vi "niFpga wdp fft sim main frame based.vi"(0 "real data in":fxp<+/-,8,1>[](array[numeric])=[0.0, 0.0], 5 "imaginary data in":fxp<+/-,8,1>[](array[numeric])=[0.0, 0.0], 9 "input frame start":bool, 12 "enable":bool) -> (3 "data indices":u16[](array[numeric]), 4 "real data out":fxp<+/-,19,2>[](array[numeric]), 6 "imaginary data out":fxp<+/-,19,2>[](array[numeric]), 10 "output valid":bool, 14 "ready for frame":bool, 15 "output frame start":bool)   [LabVIEW 2017]
uses:
  <vilib>/rvi/Analysis/measure/FFT/config/niFpgaFFTSettings.ctl
  <vilib>/rvi/Analysis/common/niLvFpgaMspClockRate.ctl
  <vilib>/rvi/Analysis/measure/FFT/config/niFpgaFFTIOPattern.ctl
  <vilib>/rvi/Analysis/measure/FFT/config/niFpgaFFTScalingScheme.ctl
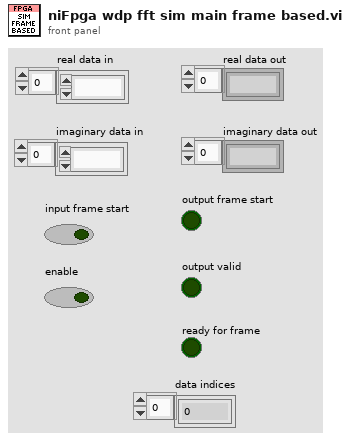
[diagram p1: front panel]
types:
  T1 = typedef "niFpgaFFTSettings.ctl" = cluster{"Number of stages":u8, "Forward?":bool, "adapt to source":bool, "Output word length":u32, "Output integer word length":i32, "Architecture":enum16{"Outside SCTL", "Inside SCTL - Burst", "Inside SCTL - Streaming"}, "input wl":u32, "input iwl":i32, "overflow?":bool, "input sign":enum32{"Signed", "Unsigned"}, "use sim models?":bool, "clock rate":T2, "pattern":T3, "mode":enum16{"Normal", "WDP"}, "scaling scheme":T4, "show enable?":bool}
  T2 = typedef "niLvFpgaMspClockRate.ctl" = enum16{"Default", "Medium", "High"}
  T3 = typedef "niFpgaFFTIOPattern.ctl" = enum16{"CI/CO", "CI/DO", "DI/CO"}
  T4 = typedef "niFpgaFFTScalingScheme.ctl" = enum16{"Unscaled", "Scaled"}
  T5 = typedef "niFpga wdp fft sim model config.ctl" = cluster{"number of stages":i32, "number of spc":i32, "Forward?":bool, "scaling scheme":T4, "internal input type":T6, "tf type":T6, "extra delay":u16, "output shift bits":i16, "reset length":u32, "input shift bits":i16, "pattern":T3}
  T6 = typedef "LVFixedPointRepBitsTypeDef.ctl" = cluster{"Signed":bool, "Word Length":u32, "Integer Word Length":i32}
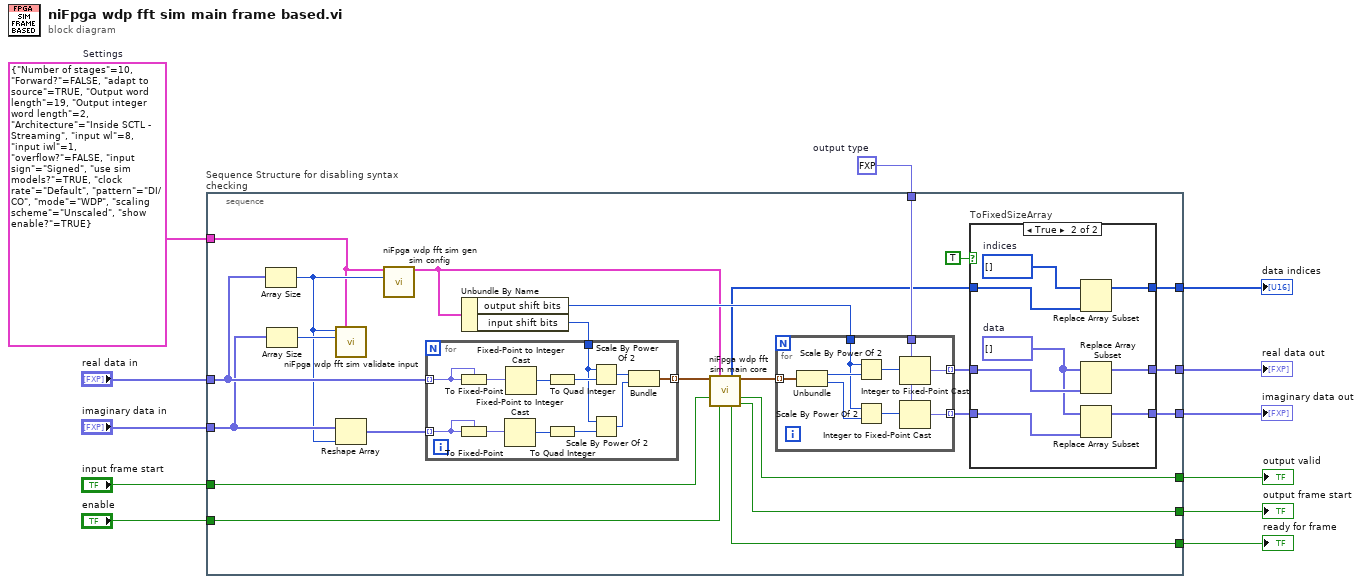
[diagram p0: block diagram]
diagram:
  w5 = fxp<+/-,19,2> 0.0  # output type
  w6 = T1 {"Number of stages"=10, "Forward?"=FALSE, "adapt to source"=TRUE, "Output word length"=19, "Output integer word length"=2, "Architecture"=enum."Inside SCTL - Streaming", "input wl"=8, "input iwl"=1, "overflow?"=FALSE, "input sign"=enum."Signed", "use sim models?"=TRUE, "clock rate"=enum."Default", "pattern"=enum."DI/CO", "mode"=enum."WDP", "scaling scheme"=enum."Unscaled", "show enable?"=TRUE}  # Settings
  n1 = stacked-sequence "Sequence Structure for disabling syntax checking" {
    tunnel: "real data in" -> [w31]
    tunnel: "imaginary data in" -> [w24]
    tunnel: "input frame start" -> [w30]
    tunnel: "enable" -> [w29]
    tunnel: [w20] -> w10
    tunnel: [w17] -> w1
    tunnel: [w16] -> w3
    tunnel: [w15] -> w9
    tunnel: [w28] -> w8
    tunnel: [w27] -> w7
    tunnel: w6 -> [w13]
    tunnel: w5 -> [w26]
    frame #0 {
      n2 = Array Size(array=w31) -> (size(s)=w22:i32)
      n3 = Array Size(array=w24) -> (size(s)=w25:i32)
      n4 = call <vilib>:"niFpga wdp fft sim validate input.vi"("size of real"=w22, "FFTConfigSettings"=w13, "size of imaginary"=w25) -> ()  [unwired: 13 in]
      n5 = Reshape Array(w24, w22) -> (w23:fxp<+/-,8,1>[])
      n6 = call <vilib>:"niFpga wdp fft sim gen sim config.vi"("FFTConfigSettings"=w13, "samples/cycle"=w22) -> ("Config"=w33:T5)  [unwired: 13 in]
      n7 = Unbundle By Name(w33) -> ("output shift bits"=w34:i16, "input shift bits"=w32:i16)
      n8 = for {
        tunnel: w31 -> [w58] mode=indexing
        tunnel: w23 -> [w60] mode=indexing
        tunnel: [w66] -> w36 mode=indexing
        tunnel: w32 -> [w63]
        n9 = To Fixed-Point(fixed-point type=w58, number=w58) -> (fixed-point=w57:fxp<+/-,8,1>)
        n10 = To Fixed-Point(fixed-point type=w60, number=w60) -> (fixed-point=w59:fxp<+/-,8,1>)
        n11 = Fixed-Point to Integer Cast(1:w59) -> (0:w67:i8)
        n12 = Fixed-Point to Integer Cast(1:w57) -> (0:w68:i8)
        n13 = To Quad Integer(1:w68) -> (0:w65:i64)
        n14 = To Quad Integer(1:w67) -> (0:w64:i64)
        n15 = Scale By Power Of 2(n=w63, x=w65) -> (x*2^n=w62:i64)
        n16 = Scale By Power Of 2(n=w63, x=w64) -> (x*2^n=w61:i64)
        n17 = Bundle(w62, w61) -> (w66:cluster{i64, i64})  [unwired: 1 in]
      }
      n18 = call <vilib>:"niFpga wdp fft sim main core.vi"("data in"=w36, "Config"=w33, "input frame start"=w30, "enable"=w29) -> ("data indices"=w21:u16[], "data out"=w35:cluster{"data re":i64, "data im":i64}[], "output valid"=w15:bool, "ready for frame"=w27:bool, "output frame start"=w28:bool)  [unwired: 7 in]
      n19 = for {
        tunnel: w26 -> [w56]
        tunnel: [w55] -> w19 mode=indexing
        tunnel: [w54] -> w18 mode=indexing
        tunnel: w34 -> [w49]
        tunnel: w35 -> [w48] mode=indexing
        n20 = Unbundle(w48) -> ("data re"=w53:i64, "data im"=w50:i64)
        n21 = Scale By Power Of 2(n=w49, x=w53) -> (x*2^n=w52:i64)
        n22 = Scale By Power Of 2(n=w49, x=w50) -> (x*2^n=w51:i64)
        n23 = Integer to Fixed-Point Cast(fixed-point type=w56, integer=w52) -> (fixed-point=w55:fxp<+/-,19,2>)
        n24 = Integer to Fixed-Point Cast(fixed-point type=w56, integer=w51) -> (fixed-point=w54:fxp<+/-,19,2>)
      }
      n25 = case "ToFixedSizeArray" shown="True" TRUE {
        tunnel: w21 -> [w39 w47]
        tunnel: [w39 w42] -> w20
        tunnel: w19 -> [w38 w46]
        tunnel: w18 -> [w37 w45]
        tunnel: [w38 w41] -> w17
        tunnel: [w37 w40] -> w16
        frame False {
        }
        frame True {
          w43 = u16[] []  # indices
          w44 = fxp<+/-,19,2>[] []  # data
          n26 = Replace Array Subset(array=w43, new element=w47) -> (w42:u16[])  [unwired: 1 in]
          n27 = Replace Array Subset(array=w44, new element=w46) -> (w41:fxp<+/-,19,2>[])  [unwired: 1 in]
          n28 = Replace Array Subset(array=w44, new element=w45) -> (w40:fxp<+/-,19,2>[])  [unwired: 1 in]
        }
      }
    }
  }
  "ready for frame" <- w7
  "output valid" <- w9
  "real data out" <- w1
  "imaginary data out" <- w3
  "output frame start" <- w8
  "data indices" <- w10
